vi "Ctor.vi"(8 "error in (no error)":errorcluster, 11 "Panel in":refnum<class "Panel.lvclass">) -> (0 "error out":errorcluster, 3 "Panel out":refnum<class "Panel.lvclass">)   [LabVIEW 2018, in "OOPanel.lvlib" / "Panel.lvclass"]
uses:
  Panel.lvclass
  Ref Data.ctl
  Panel Events.ctl
  Panel Visibility Changed.ctl
  State.ctl
  Desired Size.ctl
  Panel.lvclass/Panel.ctl
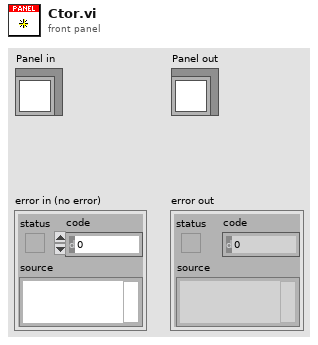
[diagram p1: front panel]
types:
  T1 = typedef "OOPanel.lvlib/Panel.lvclass/Panel Visibility Changed.ctl" = cluster{"State":T2}
  T2 = typedef "OOPanel.lvlib/Panel.lvclass/State.ctl" = enum16{"Idle", "Hidden", "Visible", "Subpanel"}
  T3 = typedef "OOPanel.lvlib/Panel.lvclass/Ref Data.ctl" = cluster{"Panel VI":refnum<vi>, "Close":bool, "Panel Events":T4, "Running":bool, "Desired Size":T5, "Subpanel":refnum<vi>, "State":T2}
  T4 = typedef "OOPanel.lvlib/Panel.lvclass/Panel Events.ctl" = cluster{"Close":refnum<user-event>, "Visibility Changed":refnum<user-event>}
  T5 = typedef "OOPanel.lvlib/Panel.lvclass/Desired Size.ctl" = cluster{"Width":i16, "Height":i16}
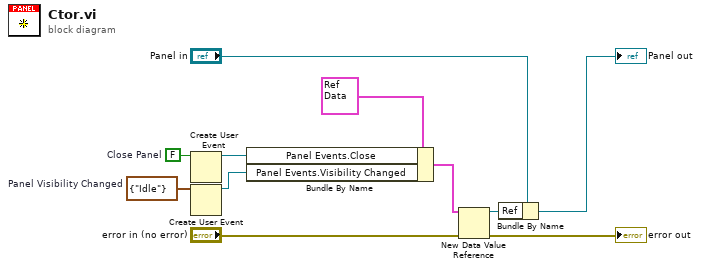
[diagram p0: block diagram]
diagram:
  w4 = T1 {"State"=enum."Idle"}  # Panel Visibility Changed
  w6 = FALSE  # Close Panel
  n1 = Create User Event(user event datatype=w6) -> (user event=w5:refnum<user-event>)  [unwired: 1 in, 1 out]
  n2 = Create User Event(user event datatype=w4) -> (user event=w3:refnum<user-event>)  [unwired: 1 in, 1 out]
  n3 = Bundle By Name(cluster=T3 {"Panel VI"=refnum, "Close"=FALSE, "Panel Events"={"Close"=refnum, "Visibility Changed"=refnum}, "Running"=FALSE, "Desired Size"={"Width"=0, "Height"=0}, "Subpanel"=refnum, "State"=enum."Idle"} ("Ref Data"), "Panel Events.Close"=w5, "Panel Events.Visibility Changed"=w3) -> (w7:T3)
  n4 = New Data Value Reference(data value=w7, error in="error in (no error)") -> (data value reference=w8:refnum<data-value>, error out=→"error out":errorcluster)
  n5 = Bundle By Name(cluster="Panel in", "Ref"=w8) -> (→"Panel out":refnum<class "Panel.lvclass">)
